vi "Untitled 2.vi"() -> ()   [LabVIEW 2024]
panel:
  in  "Array":void[](array[numeric])
  in  "Table Control":string[][](table)
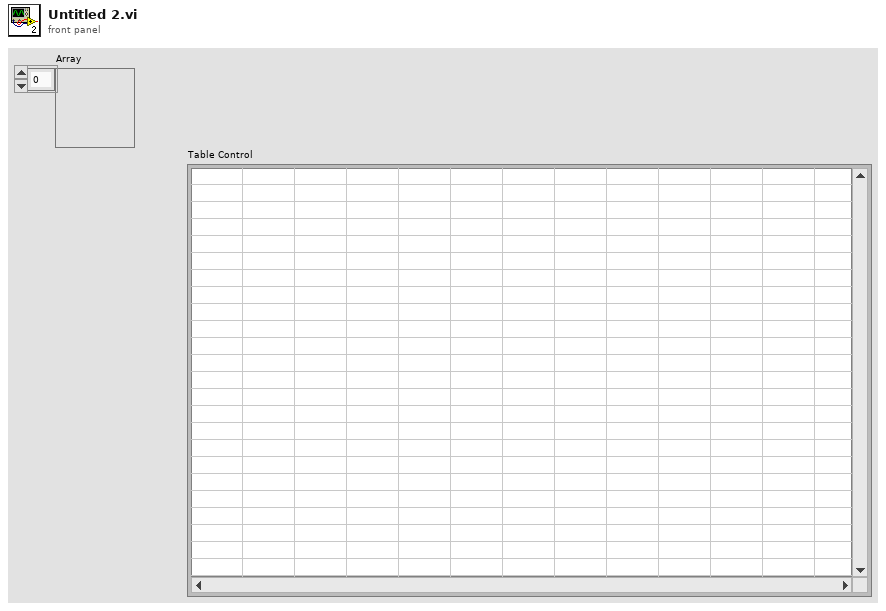
[diagram p1: front panel]
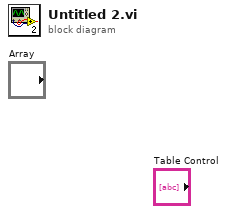
[diagram p0: block diagram]
diagram:
